vi "Increment Version Build.vi"(8 "error in (no error)":errorcluster, 10 "path":path) -> (0 "error out":errorcluster)   [LabVIEW 2019, in "VIPM.lvlib"]
uses:
  VIPM.lvlib
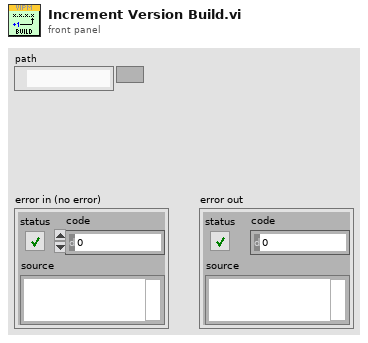
[diagram p1: front panel]
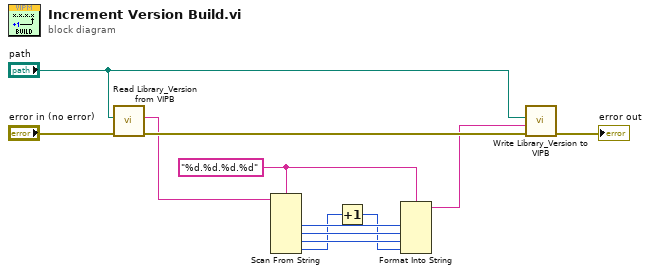
[diagram p0: block diagram]
diagram:
  w8 = "%d.%d.%d.%d" ("format string")
  n1 = call "Read Library_Version from VIPB.vi"("error in"="error in (no error)", "VIPB File Path"="path") -> ("error out"=w12:errorcluster, "Library_Version"=w5:string)  [unwired: 8 in]
  n2 = Scan From String(format string=w8, input string=w5) -> (output 1=w4:i32, output 2=w7:i32, output 3=w6:i32, output 4=w3:i32)  [unwired: 6 in, 3 out]
  n3 = Increment(x=w3) -> (x+1=w2:i32)
  n4 = Format Into String(format string=w8, w4, w7, w6, w2) -> (resulting string=w1:string)  [unwired: 2 in, 1 out]
  n5 = call "Write Library_Version to VIPB.vi"("error in"=w12, "Library_Version"=w1, "VIPB File Path"="path") -> ("error out"=→"error out":errorcluster)  [unwired: 8 in]
